vi "LuaVIEW Strip Function Name.vi"(7 "function VI name":string) -> (8 "Lua function name":string)   [LabVIEW 2013]
doc: "The name of LuaVIEW function VIs must have as format \"[re_][<table name>.]<function name>[_alternate*]_lua.vi\". This VI strips the function VI name and produces a name that can be used from within Lua. The \"_lua.vi\" postfix and any \"re_\" prefix or \"_alternate*\" infix are removed. Also, spaces are replaced by underscores. This should result in a bare function name, or a function name prefixed with a single table name. The optional \"_alternate*\" string allows multiple function VIs with the same Lua-side name to be in memory (different VIs with the same name cannot be loaded at the same time). If the VI name does not correspond to the expected format, an empty string is returned."
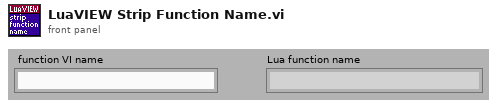
[diagram p1: front panel]
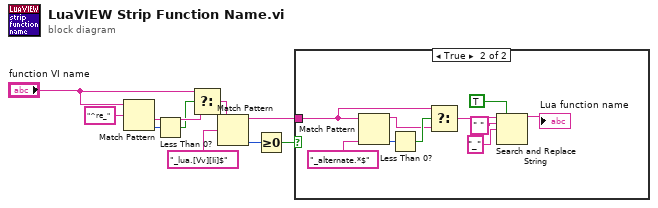
[diagram p0: block diagram]
diagram:
  n1 = Match Pattern(string="function VI name", regular expression="^re_") -> (after substring=w10:string, offset past match=w6:i32)  [unwired: 1 in, 2 out]
  n2 = Less Than 0?(x=w6) -> (x < 0?=w8:bool)
  n3 = Select(t="function VI name", s=w8, f=w10) -> (s? t:f=w9:string)
  n4 = Match Pattern(string=w9, regular expression="_lua.[Vv][Ii]$") -> (before substring=w3:string, offset past match=w2:i32)  [unwired: 1 in, 2 out]
  n5 = Greater Or Equal To 0?(x=w2) -> (x >= 0?=w1:bool)
  n6 = case shown="True" w1 {
    tunnel: w3 -> [_ w11]
    frame False {
    }
    frame True {
      n7 = Match Pattern(string=w11, regular expression="_alternate.*$") -> (before substring=w12:string, offset past match=w16:i32)  [unwired: 1 in, 2 out]
      n8 = Less Than 0?(x=w16) -> (x < 0?=w14:bool)
      n9 = Select(t=w11, s=w14, f=w12) -> (s? t:f=w13:string)
      n10 = Search and Replace String(replace all?=TRUE ("replace all? (F)"), input string=w13, search string=" ", replace string="_" ("replace string (\"\")")) -> (result string=→"Lua function name":string)  [unwired: 4 in, 3 out]
    }
  }
